vi "CRYMR_Warp_X.vi"(1 "Input":cluster{dbl, dbl}[](array[cluster]) {"?" format="%.2f"; "?" format="%.2f"}, 2 "x axis":enum32{"Linear", "Log"}(ring)) -> (0 "Output":cluster{dbl, dbl}[](array[cluster]) {"?" format="%.2f"; "?" format="%.2f"})   [LabVIEW 2013]
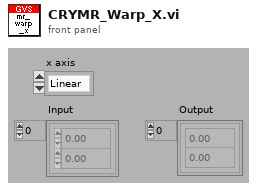
[diagram p1: front panel]
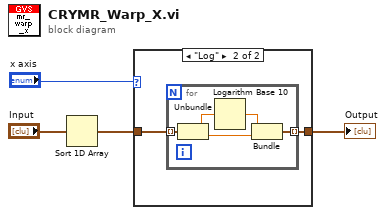
[diagram p0: block diagram]
diagram:
  n1 = Sort 1D Array(array="Input") -> (sorted array=w1:cluster{dbl, dbl}[])
  n2 = case shown="\"Log\"" "x axis" {
    tunnel: w1 -> [w5 w6]
    tunnel: [w5 w7] -> w4
    frame "Linear", Default {
    }
    frame "Log" {
      n3 = for {
        tunnel: [w12] -> w7 mode=indexing
        tunnel: w6 -> [w11] mode=indexing
        n4 = Unbundle(w11) -> (w8:dbl, w9:dbl)
        n5 = Logarithm Base 10(1:w8) -> (0:w10:dbl)
        n6 = Bundle(w10, w9) -> (w12:cluster{dbl, dbl})  [unwired: 1 out]
      }
    }
  }
  "Output" <- w4
